vi "meisterproper.vi"(1 "error in":errorcluster, 2 "mode read":i16=2, 3 "adresse":string="7") -> (0 "error out":errorcluster)   [LabVIEW 2010]
panel:
  out "status":bool
  out "data":string
  out "Numeric":i32
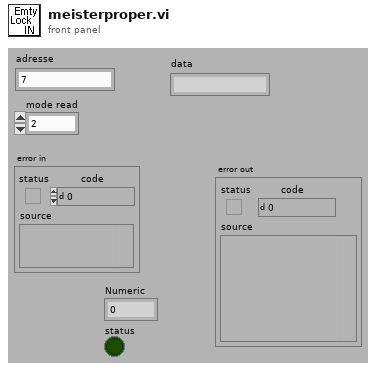
[diagram p1: front panel]
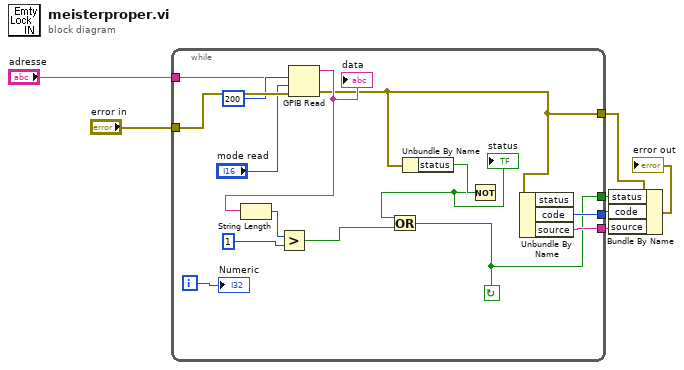
[diagram p0: block diagram]
diagram:
  n1 = while {
    tunnel: "error in" -> [w22]
    tunnel: "adresse" -> [w19]
    tunnel: [w11] -> w1
    tunnel: [w10] -> w5
    tunnel: [w9] -> w4
    tunnel: [w8] -> w3
    i -> [w16]
    stop <- w8 continue-if-true
    n2 = GPIB Read(0:w19, 1:200 ("byte count"), 2:"mode read", 3:w22) -> (5:w15:string, 7:w11:errorcluster)  [unwired: 1 in, 1 out]
    "data" <- w15
    n3 = String Length(string=w15) -> (length=w18:i32)
    n4 = Greater?(x=w18, y=1) -> (0:w13:bool)
    n5 = Unbundle By Name(w11) -> ("status"=w14:bool)
    n6 = Not(x=w14) -> (.not. x?=w12:bool)
    "status" <- w12
    n7 = Or(x=w12, y=w13) -> (x .or. y?=w8:bool)
    n8 = Unbundle By Name(w11) -> ("code"=w10:i32, "source"=w9:string)  [unwired: 1 out]
    "Numeric" <- w16
  }
  n9 = Bundle By Name(cluster=w1, "status"=w3, "code"=w5, "source"=w4) -> (→"error out":errorcluster)
